vi "zad1.vi"(9 "Numeric":u32) -> (1 "Numeric 2":i32)   [LabVIEW 2013]
uses:
  <vilib>/express/express arith-compare/Formula/XNode/ExpressFormulaBlockNode.xnode
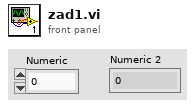
[diagram p1: front panel]
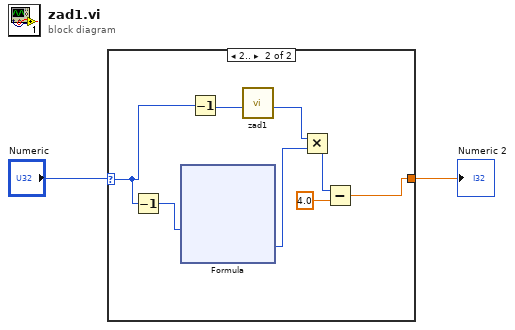
[diagram p0: block diagram]
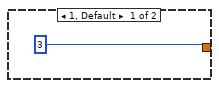
[diagram p2: hidden frame]
diagram:
  n1 = case shown="2.." "Numeric" {
    selector: "Numeric" -> [_ w4]
    tunnel: [3 w6] -> w1
    frame 1, Default {
    }
    frame 2.. {
      n2 = Decrement(x=w4) -> (x-1=w5:u32)
      n3 = xnode "Formula"("n"=w5) -> ("Result"=w10:u32)  [unwired: 1 in, 1 out]
      n4 = Decrement(x=w4) -> (x-1=w11:u32)
      n5 = call "zad1.vi"("Numeric"=w11) -> ("Numeric 2"=w9:i32)  [unwired: 10 in]
      n6 = Multiply(x=w9, y=w10) -> (x*y=w7:u32)
      n7 = Subtract(x=w7, y=4.0) -> (x-y=w6:dbl)
    }
  }
  "Numeric 2" <- w1
